vi "Boiler.vi"() -> ()   [LabVIEW 2024]
uses:
  Controls/Boiler Controls.ctl
  Controls/Boiler Simulation Controls.ctl
  Controls/Boiler Status Indicators.ctl
  Controls/eventData.ctl
  Controls/event.ctl
  Controls/controlRefs.ctl
panel:
  in  "stop":bool
  out "Boiler Status Indicators":T1={"Status"="LOCKOUT", "Primary Fan"=FALSE, "Natural Gas Valve"=FALSE, "Pilot"=FALSE, "Fuel Valve"=FALSE, "Forced Draft Fan"=FALSE, "Time Count"=0.0} {"Time Count" format="%.2g"}
  in  "Boiler Simulation Controls":T2 {"Flame Sensor Value (%)" min=0.0 max=100.0 scale=0.0..100.0}
  in  "Boiler Controls":T3 {"Fuel Valve Position" min=0.0 max=100.0 scale=0.0..100.0 scale format="%.2f"}
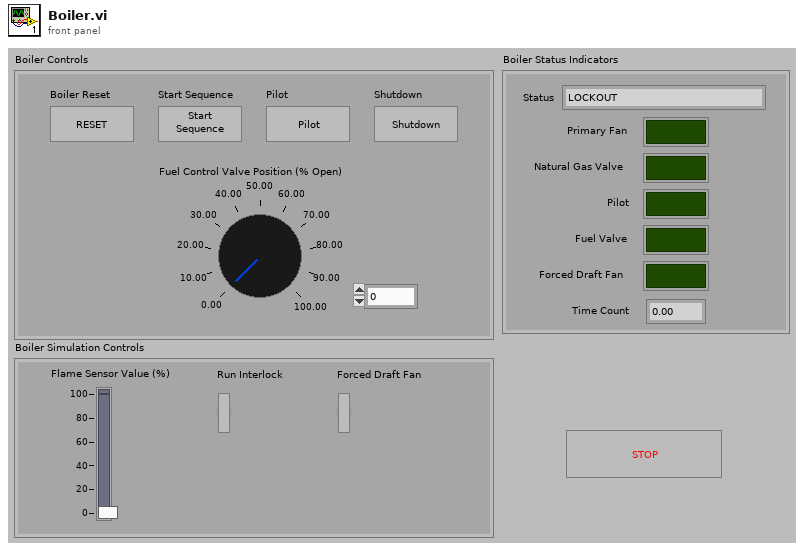
[diagram p1: front panel]
types:
  T1 = typedef "Boiler Status Indicators.ctl" = cluster{"Status":string, "Primary Fan":bool, "Natural Gas Valve":bool, "Pilot":bool, "Fuel Valve":bool, "Forced Draft Fan":bool, "Time Count":dbl}
  T2 = typedef "Boiler Simulation Controls.ctl" = cluster{"Flame Sensor Value (%)":dbl, "Run Interlock":bool, "Forced Draft Fan":bool}
  T3 = typedef "Boiler Controls.ctl" = cluster{"Boiler Reset":bool, "Start Sequence":bool, "Pilot":bool, "Shutdown":bool, "Fuel Valve Position":dbl}
  T4 = typedef "eventData.ctl" = cluster{"event":T5, "data":variant}
  T5 = typedef "event.ctl" = enum16{"appStart", "appStop", "resetLockout", "prePurge", "ignitePilot", "provePilot", "forceDraft", "startRun", "shutdownPurge", "shutdownComplete"}
  T6 = typedef "controlRefs.ctl" = cluster{"Boiler Simulation Controls":refnum<vi>, "Boiler Status Indicators":refnum<vi>, "Boiler Controls":refnum<vi>}
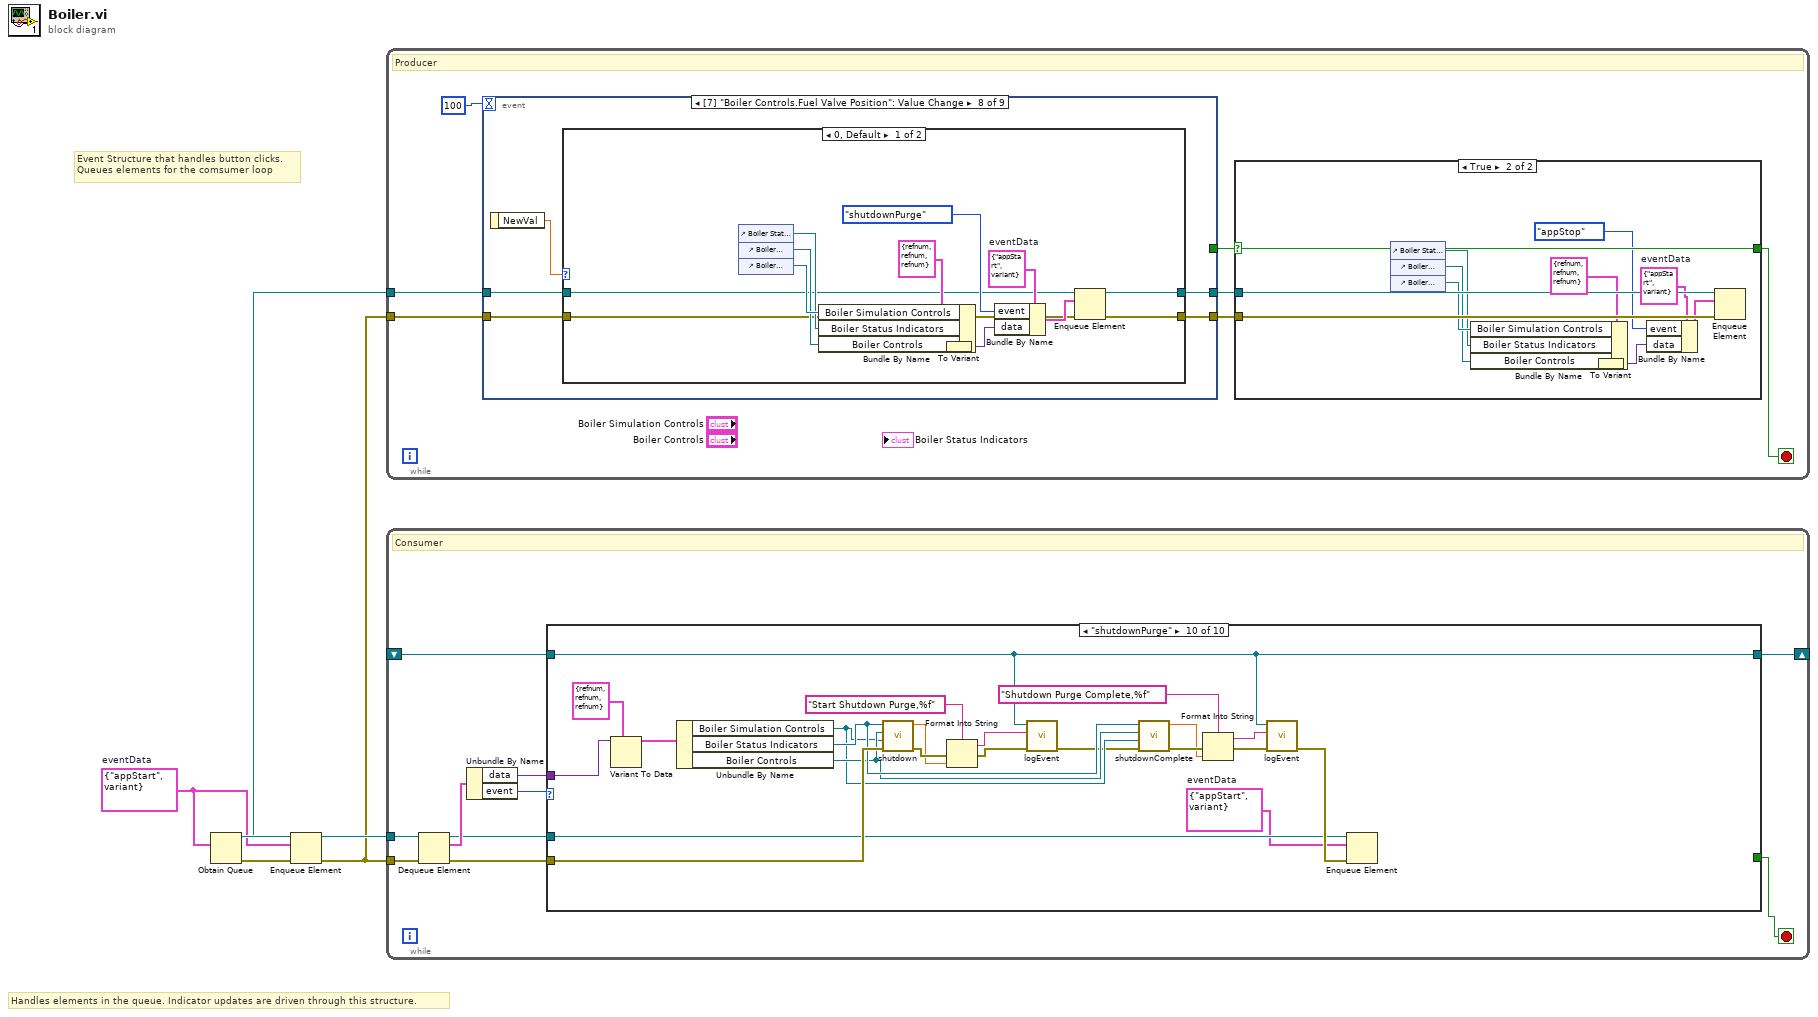
[diagram p0: block diagram]
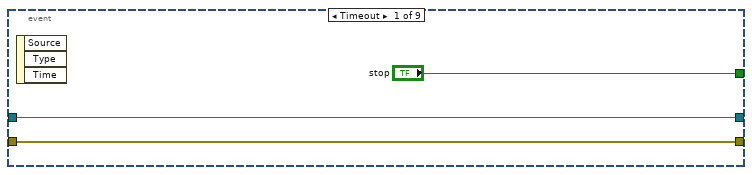
[diagram p3: hidden frame]
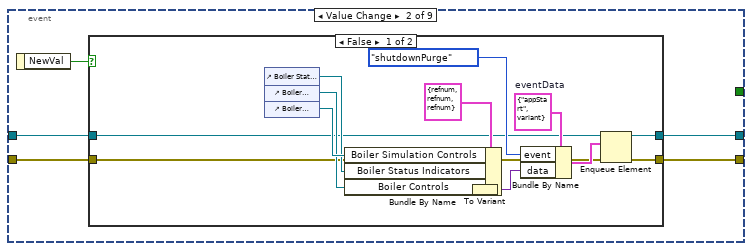
[diagram p4: hidden frame]
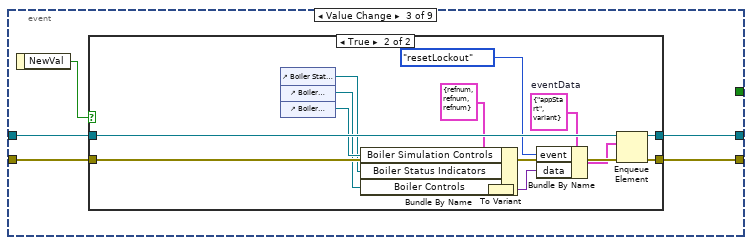
[diagram p6: hidden frame]
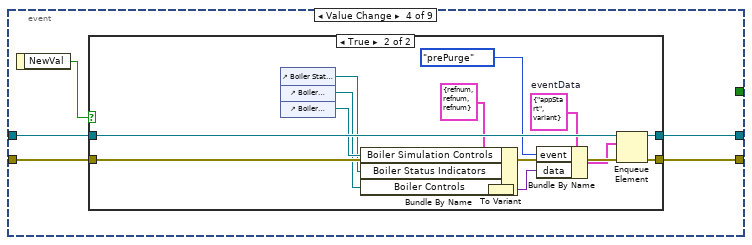
[diagram p8: hidden frame]
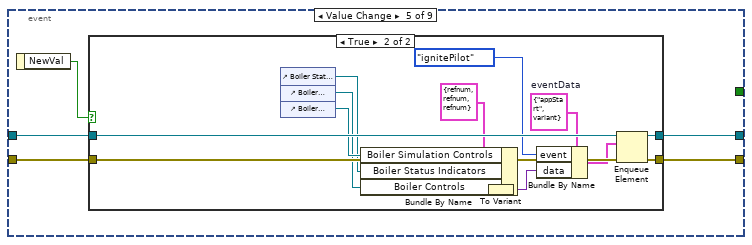
[diagram p10: hidden frame]
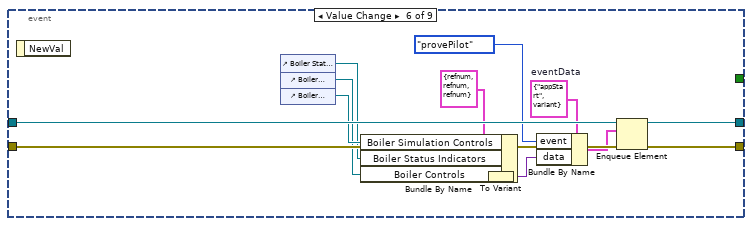
[diagram p12: hidden frame]
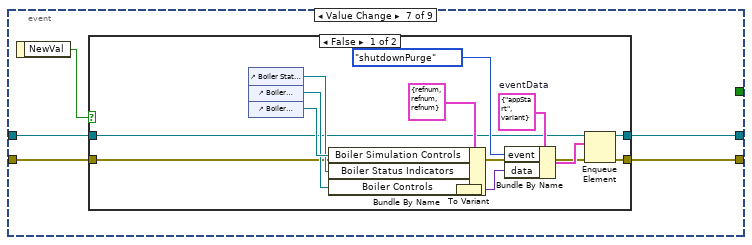
[diagram p13: hidden frame]
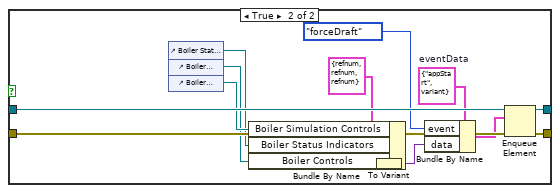
[diagram p14: hidden frame]
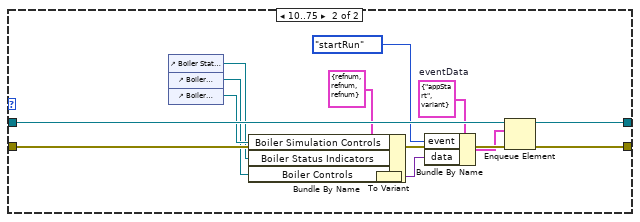
[diagram p15: hidden frame]
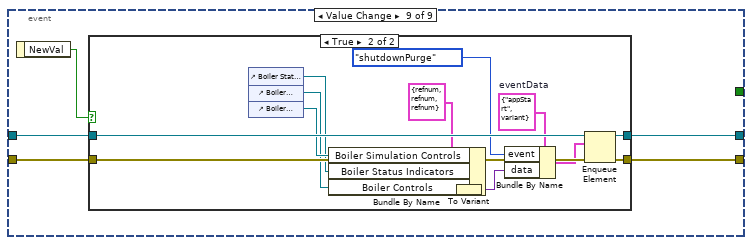
[diagram p16: hidden frame]
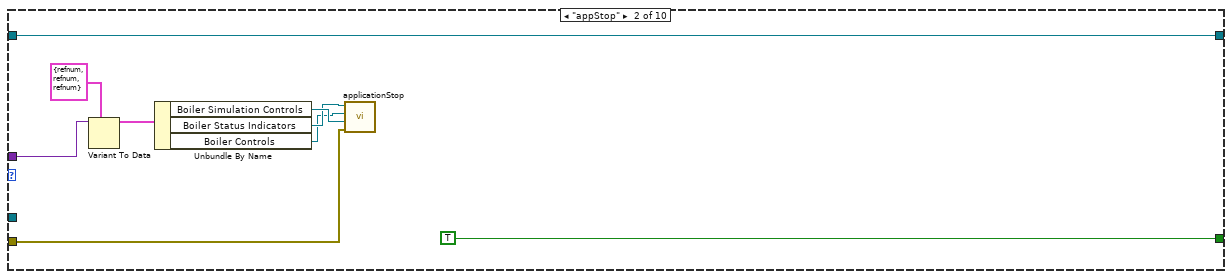
[diagram p19: hidden frame]
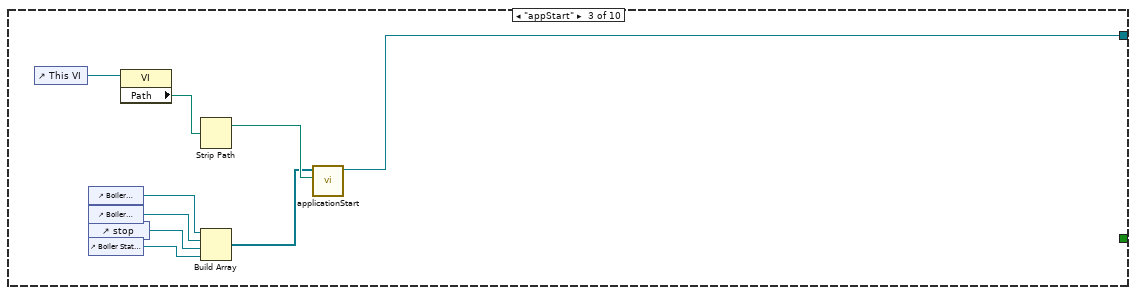
[diagram p20: hidden frame]
diagram:
  w1 = T4 {"event"=enum."appStart", "data"=variant}  # eventData
  # "Handles elements in the queue. Indicator updates are driven through this structure."
  # "Event Structure that handles button clicks.\nQueues elements for the comsumer loop"
  n1 = Obtain Queue(element data type=w1) -> (queue out=w5:refnum<queue>, error out=w4:errorcluster)  [unwired: 4 in, 1 out]
  n2 = Enqueue Element(queue=w5, element=w1, error in (no error)=w4) -> (queue out=w3:refnum<queue>, error out=w2:errorcluster)  [unwired: 1 in, 1 out]
  n3 = while {
    tunnel: w3 -> [w10]
    tunnel: w2 -> [w8]
    stop <- w6 stop-if-true
    # "Producer"
    n4 = event shown="[7] \"Boiler Controls.Fuel Valve Position\": Value Change" {
      selector: _ -> [_ _ _ _ _ _ _ _ _]
      dyn-events: _ -> [_ _ _ _ _ _ _ _ _]
      timeout: 100 -> [_ _ _ _ _ _ _ _ _]
      tunnel: ["stop" _ _ _ _ _ _ _ _] -> w11
      tunnel: w10 -> [w27 w32 w53 w73 w93 w121 w126 w157 w188]
      tunnel: [w27 w30 w51 w71 w91 w119 w124 w155 w186] -> w9
      tunnel: w8 -> [w26 w31 w52 w72 w92 w120 w125 w156 w187]
      tunnel: [w26 w29 w50 w70 w90 w118 w123 w154 w185] -> w7
      event Timeout {
        n5 = event-data() -> ()  [unwired: 1 in, 3 out]
      }
      event Value Change {
        n6 = event-data() -> ("NewVal"=w33:bool)  [unwired: 1 in]
        n7 = case shown="False" w33 {
          tunnel: w32 -> [w37 w48]
          tunnel: w31 -> [w36 w47]
          tunnel: [w35 w48] -> w30
          tunnel: [w34 w47] -> w29
          frame False {
            w39 = T4 {"event"=enum."appStart", "data"=variant}  # eventData
            n8 = control-ref of="Boiler Status Indicators"() -> (w41:refnum<vi>)
            n9 = control-ref of="Boiler Controls"() -> (w42:refnum<vi>)
            n10 = control-ref of="Boiler Simulation Controls"() -> (w43:refnum<vi>)
            n11 = Bundle By Name(cluster=T6 {"Boiler Simulation Controls"=refnum, "Boiler Status Indicators"=refnum, "Boiler Controls"=refnum} ("controlRefs"), "Boiler Simulation Controls"=w43, "Boiler Status Indicators"=w41, "Boiler Controls"=w42) -> (w44:T6)
            n12 = To Variant(anything=w44) -> (Variant=w45:variant)
            n13 = Bundle By Name(cluster=w39, "event"=event."shutdownPurge" ("element"), "data"=w45) -> (w46:T4)
            n14 = Enqueue Element(queue=w37, element=w46, error in (no error)=w36) -> (queue out=w35:refnum<queue>, error out=w34:errorcluster)  [unwired: 1 in, 1 out]
          }
          frame True {
          }
        }
      }
      event Value Change {
        n15 = event-data() -> ("NewVal"=w49:bool)  [unwired: 1 in]
        n16 = case shown="True" w49 {
          tunnel: w53 -> [w55 w68]
          tunnel: w52 -> [w54 w67]
          tunnel: [w55 w66] -> w51
          tunnel: [w54 w65] -> w50
          frame False {
          }
          frame True {
            w63 = T4 {"event"=enum."appStart", "data"=variant}  # eventData
            n17 = control-ref of="Boiler Status Indicators"() -> (w57:refnum<vi>)
            n18 = control-ref of="Boiler Controls"() -> (w58:refnum<vi>)
            n19 = control-ref of="Boiler Simulation Controls"() -> (w59:refnum<vi>)
            n20 = Bundle By Name(cluster=T6 {"Boiler Simulation Controls"=refnum, "Boiler Status Indicators"=refnum, "Boiler Controls"=refnum} ("controlRefs"), "Boiler Simulation Controls"=w59, "Boiler Status Indicators"=w57, "Boiler Controls"=w58) -> (w61:T6)
            n21 = To Variant(anything=w61) -> (Variant=w62:variant)
            n22 = Bundle By Name(cluster=w63, "event"=event."resetLockout" ("element"), "data"=w62) -> (w64:T4)
            n23 = Enqueue Element(queue=w68, element=w64, error in (no error)=w67) -> (queue out=w66:refnum<queue>, error out=w65:errorcluster)  [unwired: 1 in, 1 out]
          }
        }
      }
      event Value Change {
        n24 = event-data() -> ("NewVal"=w69:bool)  [unwired: 1 in]
        n25 = case shown="True" w69 {
          tunnel: w73 -> [w75 w88]
          tunnel: w72 -> [w74 w87]
          tunnel: [w75 w86] -> w71
          tunnel: [w74 w85] -> w70
          frame False {
          }
          frame True {
            w83 = T4 {"event"=enum."appStart", "data"=variant}  # eventData
            n26 = control-ref of="Boiler Status Indicators"() -> (w77:refnum<vi>)
            n27 = control-ref of="Boiler Controls"() -> (w78:refnum<vi>)
            n28 = control-ref of="Boiler Simulation Controls"() -> (w79:refnum<vi>)
            n29 = Bundle By Name(cluster=T6 {"Boiler Simulation Controls"=refnum, "Boiler Status Indicators"=refnum, "Boiler Controls"=refnum} ("controlRefs"), "Boiler Simulation Controls"=w79, "Boiler Status Indicators"=w77, "Boiler Controls"=w78) -> (w81:T6)
            n30 = To Variant(anything=w81) -> (Variant=w82:variant)
            n31 = Bundle By Name(cluster=w83, "event"=event."prePurge" ("element"), "data"=w82) -> (w84:T4)
            n32 = Enqueue Element(queue=w88, element=w84, error in (no error)=w87) -> (queue out=w86:refnum<queue>, error out=w85:errorcluster)  [unwired: 1 in, 1 out]
          }
        }
      }
      event Value Change {
        n33 = event-data() -> ("NewVal"=w89:bool)  [unwired: 1 in]
        n34 = case shown="True" w89 {
          tunnel: w93 -> [w95 w108]
          tunnel: w92 -> [w94 w107]
          tunnel: [w95 w106] -> w91
          tunnel: [w94 w105] -> w90
          frame False {
          }
          frame True {
            w103 = T4 {"event"=enum."appStart", "data"=variant}  # eventData
            n35 = control-ref of="Boiler Status Indicators"() -> (w97:refnum<vi>)
            n36 = control-ref of="Boiler Controls"() -> (w98:refnum<vi>)
            n37 = control-ref of="Boiler Simulation Controls"() -> (w99:refnum<vi>)
            n38 = Bundle By Name(cluster=T6 {"Boiler Simulation Controls"=refnum, "Boiler Status Indicators"=refnum, "Boiler Controls"=refnum} ("controlRefs"), "Boiler Simulation Controls"=w99, "Boiler Status Indicators"=w97, "Boiler Controls"=w98) -> (w101:T6)
            n39 = To Variant(anything=w101) -> (Variant=w102:variant)
            n40 = Bundle By Name(cluster=w103, "event"=event."ignitePilot" ("element"), "data"=w102) -> (w104:T4)
            n41 = Enqueue Element(queue=w108, element=w104, error in (no error)=w107) -> (queue out=w106:refnum<queue>, error out=w105:errorcluster)  [unwired: 1 in, 1 out]
          }
        }
      }
      event Value Change {
        w116 = T4 {"event"=enum."appStart", "data"=variant}  # eventData
        n42 = event-data() -> ()  [unwired: 1 in, 1 out]
        n43 = control-ref of="Boiler Status Indicators"() -> (w110:refnum<vi>)
        n44 = control-ref of="Boiler Controls"() -> (w111:refnum<vi>)
        n45 = control-ref of="Boiler Simulation Controls"() -> (w112:refnum<vi>)
        n46 = Bundle By Name(cluster=T6 {"Boiler Simulation Controls"=refnum, "Boiler Status Indicators"=refnum, "Boiler Controls"=refnum} ("controlRefs"), "Boiler Simulation Controls"=w112, "Boiler Status Indicators"=w110, "Boiler Controls"=w111) -> (w114:T6)
        n47 = To Variant(anything=w114) -> (Variant=w115:variant)
        n48 = Bundle By Name(cluster=w116, "event"=event."provePilot" ("element"), "data"=w115) -> (w117:T4)
        n49 = Enqueue Element(queue=w121, element=w117, error in (no error)=w120) -> (queue out=w119:refnum<queue>, error out=w118:errorcluster)  [unwired: 1 in, 1 out]
      }
      event Value Change {
        n50 = event-data() -> ("NewVal"=w122:bool)  [unwired: 1 in]
        n51 = case shown="False" w122 {
          tunnel: w126 -> [w130 w152]
          tunnel: w125 -> [w129 w151]
          tunnel: [w127 w150] -> w124
          tunnel: [w128 w149] -> w123
          frame False {
            w132 = T4 {"event"=enum."appStart", "data"=variant}  # eventData
            n52 = control-ref of="Boiler Status Indicators"() -> (w134:refnum<vi>)
            n53 = control-ref of="Boiler Controls"() -> (w135:refnum<vi>)
            n54 = control-ref of="Boiler Simulation Controls"() -> (w136:refnum<vi>)
            n55 = Bundle By Name(cluster=T6 {"Boiler Simulation Controls"=refnum, "Boiler Status Indicators"=refnum, "Boiler Controls"=refnum} ("controlRefs"), "Boiler Simulation Controls"=w136, "Boiler Status Indicators"=w134, "Boiler Controls"=w135) -> (w137:T6)
            n56 = To Variant(anything=w137) -> (Variant=w138:variant)
            n57 = Bundle By Name(cluster=w132, "event"=event."shutdownPurge" ("element"), "data"=w138) -> (w139:T4)
            n58 = Enqueue Element(queue=w130, element=w139, error in (no error)=w129) -> (queue out=w127:refnum<queue>, error out=w128:errorcluster)  [unwired: 1 in, 1 out]
          }
          frame True {
            w147 = T4 {"event"=enum."appStart", "data"=variant}  # eventData
            n59 = control-ref of="Boiler Status Indicators"() -> (w141:refnum<vi>)
            n60 = control-ref of="Boiler Controls"() -> (w142:refnum<vi>)
            n61 = control-ref of="Boiler Simulation Controls"() -> (w143:refnum<vi>)
            n62 = Bundle By Name(cluster=T6 {"Boiler Simulation Controls"=refnum, "Boiler Status Indicators"=refnum, "Boiler Controls"=refnum} ("controlRefs"), "Boiler Simulation Controls"=w143, "Boiler Status Indicators"=w141, "Boiler Controls"=w142) -> (w145:T6)
            n63 = To Variant(anything=w145) -> (Variant=w146:variant)
            n64 = Bundle By Name(cluster=w147, "event"=event."forceDraft" ("element"), "data"=w146) -> (w148:T4)
            n65 = Enqueue Element(queue=w152, element=w148, error in (no error)=w151) -> (queue out=w150:refnum<queue>, error out=w149:errorcluster)  [unwired: 1 in, 1 out]
          }
        }
      }
      event Value Change {
        n66 = event-data() -> ("NewVal"=w153:dbl)  [unwired: 1 in]
        n67 = case shown="0, Default" w153 {
          tunnel: w157 -> [w160 w183]
          tunnel: w156 -> [w161 w182]
          tunnel: [w159 w181] -> w155
          tunnel: [w158 w180] -> w154
          frame 0, Default {
            w169 = T4 {"event"=enum."appStart", "data"=variant}  # eventData
            n68 = control-ref of="Boiler Status Indicators"() -> (w163:refnum<vi>)
            n69 = control-ref of="Boiler Controls"() -> (w164:refnum<vi>)
            n70 = control-ref of="Boiler Simulation Controls"() -> (w165:refnum<vi>)
            n71 = Bundle By Name(cluster=T6 {"Boiler Simulation Controls"=refnum, "Boiler Status Indicators"=refnum, "Boiler Controls"=refnum} ("controlRefs"), "Boiler Simulation Controls"=w165, "Boiler Status Indicators"=w163, "Boiler Controls"=w164) -> (w167:T6)
            n72 = To Variant(anything=w167) -> (Variant=w168:variant)
            n73 = Bundle By Name(cluster=w169, "event"=event."shutdownPurge" ("element"), "data"=w168) -> (w170:T4)
            n74 = Enqueue Element(queue=w160, element=w170, error in (no error)=w161) -> (queue out=w159:refnum<queue>, error out=w158:errorcluster)  [unwired: 1 in, 1 out]
          }
          frame 10..75 {
            w178 = T4 {"event"=enum."appStart", "data"=variant}  # eventData
            n75 = control-ref of="Boiler Status Indicators"() -> (w172:refnum<vi>)
            n76 = control-ref of="Boiler Controls"() -> (w173:refnum<vi>)
            n77 = control-ref of="Boiler Simulation Controls"() -> (w174:refnum<vi>)
            n78 = Bundle By Name(cluster=T6 {"Boiler Simulation Controls"=refnum, "Boiler Status Indicators"=refnum, "Boiler Controls"=refnum} ("controlRefs"), "Boiler Simulation Controls"=w174, "Boiler Status Indicators"=w172, "Boiler Controls"=w173) -> (w176:T6)
            n79 = To Variant(anything=w176) -> (Variant=w177:variant)
            n80 = Bundle By Name(cluster=w178, "event"=event."startRun" ("element"), "data"=w177) -> (w179:T4)
            n81 = Enqueue Element(queue=w183, element=w179, error in (no error)=w182) -> (queue out=w181:refnum<queue>, error out=w180:errorcluster)  [unwired: 1 in, 1 out]
          }
        }
      }
      event Value Change {
        n82 = event-data() -> ("NewVal"=w184:bool)  [unwired: 1 in]
        n83 = case shown="True" w184 {
          tunnel: w188 -> [w190 w203]
          tunnel: w187 -> [w189 w202]
          tunnel: [w190 w201] -> w186
          tunnel: [w189 w200] -> w185
          frame False {
          }
          frame True {
            w198 = T4 {"event"=enum."appStart", "data"=variant}  # eventData
            n84 = control-ref of="Boiler Status Indicators"() -> (w192:refnum<vi>)
            n85 = control-ref of="Boiler Controls"() -> (w193:refnum<vi>)
            n86 = control-ref of="Boiler Simulation Controls"() -> (w194:refnum<vi>)
            n87 = Bundle By Name(cluster=T6 {"Boiler Simulation Controls"=refnum, "Boiler Status Indicators"=refnum, "Boiler Controls"=refnum} ("controlRefs"), "Boiler Simulation Controls"=w194, "Boiler Status Indicators"=w192, "Boiler Controls"=w193) -> (w196:T6)
            n88 = To Variant(anything=w196) -> (Variant=w197:variant)
            n89 = Bundle By Name(cluster=w198, "event"=event."shutdownPurge" ("element"), "data"=w197) -> (w199:T4)
            n90 = Enqueue Element(queue=w203, element=w199, error in (no error)=w202) -> (queue out=w201:refnum<queue>, error out=w200:errorcluster)  [unwired: 1 in, 1 out]
          }
        }
      }
    }
    n91 = case shown="True" w11 {
      selector: w11 -> [w13 w23]
      tunnel: w9 -> [_ w25]
      tunnel: w7 -> [_ w24]
      tunnel: [w13 w23] -> w6
      frame False {
      }
      frame True {
        w16 = T4 {"event"=enum."appStart", "data"=variant}  # eventData
        n92 = control-ref of="Boiler Status Indicators"() -> (w18:refnum<vi>)
        n93 = control-ref of="Boiler Controls"() -> (w19:refnum<vi>)
        n94 = control-ref of="Boiler Simulation Controls"() -> (w20:refnum<vi>)
        n95 = Bundle By Name(cluster=T6 {"Boiler Simulation Controls"=refnum, "Boiler Status Indicators"=refnum, "Boiler Controls"=refnum} ("controlRefs"), "Boiler Simulation Controls"=w20, "Boiler Status Indicators"=w18, "Boiler Controls"=w19) -> (w21:T6)
        n96 = To Variant(anything=w21) -> (Variant=w22:variant)
        n97 = Bundle By Name(cluster=w16, "event"=event."appStop" ("element"), "data"=w22) -> (w14:T4)
        n98 = Enqueue Element(queue=w25, element=w14, error in (no error)=w24) -> ()  [unwired: 1 in, 3 out]
      }
    }
  }
  n99 = while {
    tunnel: w3 -> [w213]
    tunnel: w2 -> [w212]
    shift-right: [w207] -> _
    shift-left: _ -> [w206]
    stop <- w211 stop-if-true
    # "Consumer"
    n100 = Dequeue Element(queue=w213, error in (no error)=w212) -> (queue out=w204:refnum<queue>, element=w210:T4, error out=w205:errorcluster)  [unwired: 1 in, 1 out]
    n101 = Unbundle By Name(w210) -> ("data"=w208:variant, "event"=w209:T5)
    n102 = case shown="\"shutdownPurge\"" w209 {
      tunnel: [_ TRUE _ _ _ _ _ _ _ _] -> w211
      tunnel: w208 -> [_ w219 _ w241 w261 w271 w287 w297 w310 w332]
      tunnel: [w214 w222 w224 w233 w245 w265 w277 w295 w305 w321] -> w207
      tunnel: w206 -> [w214 w222 _ w233 w245 w265 w277 w295 w305 w321]
      tunnel: w205 -> [_ w218 _ _ w260 w270 w283 w296 w306 w331]
      tunnel: w204 -> [_ _ _ _ _ _ _ _ _ w314]
      frame Default {
      }
      frame "appStop" {
        n103 = Variant To Data(type=T6 {"Boiler Simulation Controls"=refnum, "Boiler Status Indicators"=refnum, "Boiler Controls"=refnum} ("controlRefs"), Variant=w219) -> (data=w220:T6)  [unwired: 1 in, 1 out]
        n104 = Unbundle By Name(w220) -> ("Boiler Simulation Controls"=w217:refnum<vi>, "Boiler Status Indicators"=w216:refnum<vi>, "Boiler Controls"=w215:refnum<vi>)
        n105 = call "applicationStop.vi"("error in"=w218, "Boiler Simulation Controls"=w217, "Boiler Controls"=w215, "Boiler Status Indicators"=w216) -> ()  [unwired: 7 in, 1 out]
      }
      frame "appStart" {
        n106 = control-ref of="This VI"() -> (w227:refnum<vi>)
        n107 = control-ref of="Boiler Controls"() -> (w228:refnum<vi>)
        n108 = control-ref of="Boiler Simulation Controls"() -> (w229:refnum<vi>)
        n109 = control-ref of="stop"() -> (w230:refnum<vi>)
        n110 = control-ref of="Boiler Status Indicators"() -> (w231:refnum<vi>)
        n111 = property class="VI"(reference=w227) -> ("Path"=w232:path)  [unwired: 1 in, 2 out]
        n112 = Strip Path(path=w232) -> (stripped path=w226:path)  [unwired: 1 out]
        n113 = Build Array(w228, w229, w230, w231) -> (w225:refnum<vi>[])
        n114 = call "applicationStart.vi"("File Path"=w226, "controlsArray"=w225) -> ("fileRef"=w224:refnum<file>)  [unwired: 8 in, 1 out]
      }
      frame "resetLockout" {
        n115 = Variant To Data(type=T6 {"Boiler Simulation Controls"=refnum, "Boiler Status Indicators"=refnum, "Boiler Controls"=refnum} ("controlRefs"), Variant=w241) -> (data=w239:T6)  [unwired: 1 in, 1 out]
        n116 = Unbundle By Name(w239) -> ("Boiler Simulation Controls"=w238:refnum<vi>, "Boiler Status Indicators"=w237:refnum<vi>, "Boiler Controls"=w236:refnum<vi>)
        n117 = call "resetLockout.vi"("Boiler Simulation Controls"=w238, "Boiler Controls"=w236, "Boiler Status Indicators"=w237) -> ("error out"=w235:errorcluster, "Ready?"=w234:bool)  [unwired: 7 in]
        n118 = case shown="True" w234 {
          tunnel: w235 -> [_ w244]
          tunnel: w233 -> [_ w243]
          frame False {
          }
          frame True {
            n119 = call "logEvent.vi"("error in"=w244, "event,data"="Boiler Ready,0", "fileRef"=w243) -> ()  [unwired: 8 in, 1 out]
          }
        }
      }
      frame "prePurge" {
        n120 = Variant To Data(type=T6 {"Boiler Simulation Controls"=refnum, "Boiler Status Indicators"=refnum, "Boiler Controls"=refnum} ("controlRefs"), Variant=w261) -> (data=w262:T6)  [unwired: 1 in, 1 out]
        n121 = Unbundle By Name(w262) -> ("Boiler Simulation Controls"=w250:refnum<vi>, "Boiler Status Indicators"=w251:refnum<vi>, "Boiler Controls"=w252:refnum<vi>)
        n122 = call "prePurge.vi"("error in"=w260, "Boiler Simulation Controls"=w250, "Boiler Controls"=w252, "Boiler Status Indicators"=w251) -> ("error out"=w259:errorcluster, "elapsedTime"=w257:dbl)  [unwired: 6 in]
        n123 = Format Into String(format string="Start Pre-Purge,%f" ("event,data"), error in=w259, w257) -> (resulting string=w255:string, error out=w258:errorcluster)  [unwired: 1 in]
        n124 = call "logEvent.vi"("error in"=w258, "event,data"=w255, "fileRef"=w245) -> ("error out"=w254:errorcluster)  [unwired: 8 in]
        n125 = call "prePurge2.vi"("error in"=w254, "Boiler Simulation Controls"=w250, "Boiler Controls"=w252, "Boiler Status Indicators"=w251) -> ("error out"=w253:errorcluster, "elapsedTime"=w248:dbl)  [unwired: 6 in]
        n126 = Format Into String(format string="Pre-Purge Complete,%f" ("event,data"), error in=w253, w248) -> (resulting string=w246:string, error out=w247:errorcluster)  [unwired: 1 in]
        n127 = call "logEvent.vi"("error in"=w247, "event,data"=w246, "fileRef"=w245) -> ()  [unwired: 8 in, 1 out]
      }
      frame "ignitePilot" {
        n128 = Variant To Data(type=T6 {"Boiler Simulation Controls"=refnum, "Boiler Status Indicators"=refnum, "Boiler Controls"=refnum} ("controlRefs"), Variant=w271) -> (data=w273:T6)  [unwired: 1 in, 1 out]
        n129 = Unbundle By Name(w273) -> ("Boiler Simulation Controls"=w268:refnum<vi>, "Boiler Status Indicators"=w267:refnum<vi>, "Boiler Controls"=w269:refnum<vi>)
        n130 = call "ignitePilot.vi"("error in"=w270, "Boiler Simulation Controls"=w268, "Boiler Controls"=w269, "Boiler Status Indicators"=w267) -> ("error out"=w266:errorcluster, "pilotOn?"=w264:bool)  [unwired: 6 in]
        n131 = case shown="True" w264 {
          tunnel: w266 -> [_ w276]
          tunnel: w265 -> [_ w275]
          frame False {
          }
          frame True {
            n132 = call "logEvent.vi"("error in"=w276, "event,data"="Pilot ON,True", "fileRef"=w275) -> ()  [unwired: 8 in, 1 out]
          }
        }
      }
      frame "provePilot" {
        n133 = Variant To Data(type=T6 {"Boiler Simulation Controls"=refnum, "Boiler Status Indicators"=refnum, "Boiler Controls"=refnum} ("controlRefs"), Variant=w287) -> (data=w289:T6)  [unwired: 1 in, 1 out]
        n134 = Unbundle By Name(w289) -> ("Boiler Simulation Controls"=w284:refnum<vi>, "Boiler Status Indicators"=w286:refnum<vi>, "Boiler Controls"=w285:refnum<vi>)
        n135 = call "provePilot.vi"("error in"=w283, "Boiler Simulation Controls"=w284, "Boiler Controls"=w285, "Boiler Status Indicators"=w286) -> ("error out"=w279:errorcluster, "sensor"=w278:dbl)  [unwired: 6 in]
        n136 = Format Into String(format string="Pilot Proved,%f" ("event,data"), error in=w279, w278) -> (resulting string=w280:string, error out=w281:errorcluster)  [unwired: 1 in]
        n137 = call "logEvent.vi"("error in"=w281, "event,data"=w280, "fileRef"=w277) -> ()  [unwired: 8 in, 1 out]
      }
      frame "forceDraft" {
        n138 = Variant To Data(type=T6 {"Boiler Simulation Controls"=refnum, "Boiler Status Indicators"=refnum, "Boiler Controls"=refnum} ("controlRefs"), Variant=w297) -> (data=w299:T6)  [unwired: 1 in, 1 out]
        n139 = Unbundle By Name(w299) -> ("Boiler Simulation Controls"=w291:refnum<vi>, "Boiler Status Indicators"=w293:refnum<vi>, "Boiler Controls"=w292:refnum<vi>)
        n140 = call "startRun1.vi"("error in"=w296, "Boiler Simulation Controls"=w291, "Boiler Controls"=w292, "Boiler Status Indicators"=w293) -> ("error out"=w290:errorcluster)  [unwired: 7 in]
        n141 = call "logEvent.vi"("error in"=w290, "event,data"="Forced Draft-Fan ON,True", "fileRef"=w295) -> ()  [unwired: 8 in, 1 out]
      }
      frame "startRun" {
        n142 = Variant To Data(type=T6 {"Boiler Simulation Controls"=refnum, "Boiler Status Indicators"=refnum, "Boiler Controls"=refnum} ("controlRefs"), Variant=w310) -> (data=w312:T6)  [unwired: 1 in, 1 out]
        n143 = Unbundle By Name(w312) -> ("Boiler Simulation Controls"=w307:refnum<vi>, "Boiler Status Indicators"=w308:refnum<vi>, "Boiler Controls"=w309:refnum<vi>)
        n144 = call "startRun2.vi"("error in"=w306, "Boiler Simulation Controls"=w307, "Boiler Controls"=w309, "Boiler Status Indicators"=w308) -> ("error out"=w303:errorcluster, "Fuel Valve Position"=w301:dbl)  [unwired: 6 in]
        n145 = Format Into String(format string="Boiler Running,%f" ("event,data"), error in=w303, w301) -> (resulting string=w300:string, error out=w302:errorcluster)  [unwired: 1 in]
        n146 = call "logEvent.vi"("error in"=w302, "event,data"=w300, "fileRef"=w305) -> ()  [unwired: 8 in, 1 out]
      }
      frame "shutdownPurge" {
        w313 = T4 {"event"=enum."appStart", "data"=variant}  # eventData
        n147 = Variant To Data(type=T6 {"Boiler Simulation Controls"=refnum, "Boiler Status Indicators"=refnum, "Boiler Controls"=refnum} ("controlRefs"), Variant=w332) -> (data=w334:T6)  [unwired: 1 in, 1 out]
        n148 = Unbundle By Name(w334) -> ("Boiler Simulation Controls"=w323:refnum<vi>, "Boiler Status Indicators"=w325:refnum<vi>, "Boiler Controls"=w324:refnum<vi>)
        n149 = call "shutdown.vi"("error in"=w331, "Boiler Simulation Controls"=w323, "Boiler Controls"=w324, "Boiler Status Indicators"=w325) -> ("error out"=w329:errorcluster, "elapsedTime"=w327:dbl)  [unwired: 6 in]
        n150 = Format Into String(format string="Start Shutdown Purge,%f" ("event,data"), error in=w329, w327) -> (resulting string=w326:string, error out=w328:errorcluster)  [unwired: 1 in]
        n151 = call "logEvent.vi"("error in"=w328, "event,data"=w326, "fileRef"=w321) -> ("error out"=w322:errorcluster)  [unwired: 8 in]
        n152 = call "shutdownComplete.vi"("error in"=w322, "Boiler Simulation Controls"=w323, "Boiler Controls"=w324, "Boiler Status Indicators"=w325) -> ("error out"=w320:errorcluster, "elapsedTime"=w318:dbl)  [unwired: 6 in]
        n153 = Format Into String(format string="Shutdown Purge Complete,%f" ("event,data"), error in=w320, w318) -> (resulting string=w316:string, error out=w319:errorcluster)  [unwired: 1 in]
        n154 = call "logEvent.vi"("error in"=w319, "event,data"=w316, "fileRef"=w321) -> ("error out"=w315:errorcluster)  [unwired: 8 in]
        n155 = Enqueue Element(queue=w314, element=w313, error in (no error)=w315) -> ()  [unwired: 1 in, 3 out]
      }
    }
  }
